vi "StartAcq.vi"(6 "LabVIEW Web Service Request":refnum<class "Web Request.lvclass">) -> ()   [LabVIEW 2017]
doc: "StartAcq POST method receives JSON string with StartAcq boolean value, and saves it into shared variable."
uses:
  <vilib>/wsapi/Web Request.lvclass
panel:
  out "Start Acq":bool
  # "Use the Web Service Request input terminal to call the VIs on the Web Services palette. Do not remove it from the connector pane unless you don't need access to the palette."
  # "Each additional control wired to the connector pane will be available as an input in the URL. To include an indicator in terminal-mode output (the default setting), it must also be wired to the connector pane."
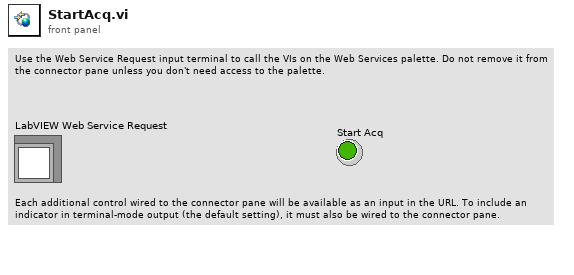
[diagram p1: front panel]
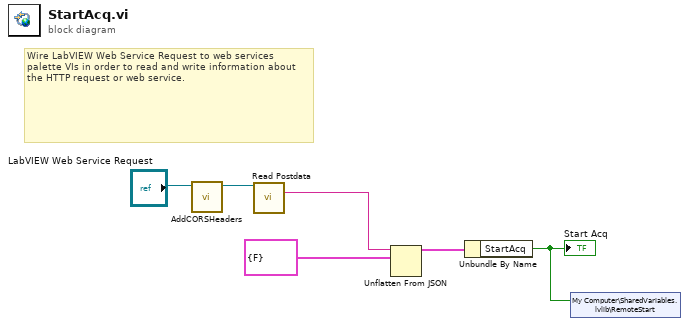
[diagram p0: block diagram]
diagram:
  # "Wire LabVIEW Web Service Request to web services palette VIs in order to read and write information about the HTTP request or web service."
  n1 = call "AddCORSHeaders.vi"("Web Request in"="LabVIEW Web Service Request") -> ("Web Request out"=w2:refnum<class "Web Request.lvclass">)  [unwired: 10 in]
  n2 = call <vilib>:"Read Postdata.vi"("LabVIEW Web Service Request"=w2) -> ("postdata"=w6:string)  [unwired: 12 in, 2 out]
  n3 = Unflatten From JSON(JSON string=w6, type and defaults=cluster{"StartAcq":bool} {"StartAcq"=FALSE}) -> (value=w5:cluster{"StartAcq":bool})  [unwired: 5 in, 1 out]
  n4 = Unbundle By Name(w5) -> ("StartAcq"=w1:bool)
  "Start Acq" <- w1
  n5 = shared-variable "My Computer\\SharedVariables.lvlib\\RemoteStart"(w1) -> ()  [unwired: 1 in, 1 out]
